vi "Softplus.vi"(2 "Z":dbl) -> (0 "Softplus(Z)":dbl)   [LabVIEW 2020]
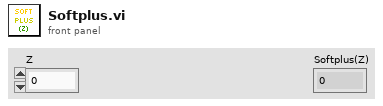
[diagram p1: front panel]
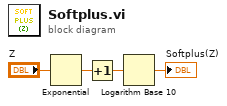
[diagram p0: block diagram]
diagram:
  n1 = Exponential(1:"Z") -> (0:w2:dbl)
  n2 = Increment(x=w2) -> (x+1=w1:dbl)
  n3 = Logarithm Base 10(1:w1) -> (0:→"Softplus(Z)":dbl)
